vi "String.Validate IP Address String.vi"(11 "IP Address":string) -> (3 "Valid":bool)   [LabVIEW 2019]
panel:
  out "Val 4":i32
  out "Val 3":i32
  out "Val 2":i32
  out "Val 1":i32
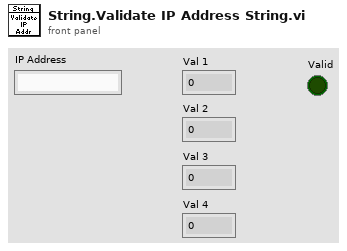
[diagram p1: front panel]
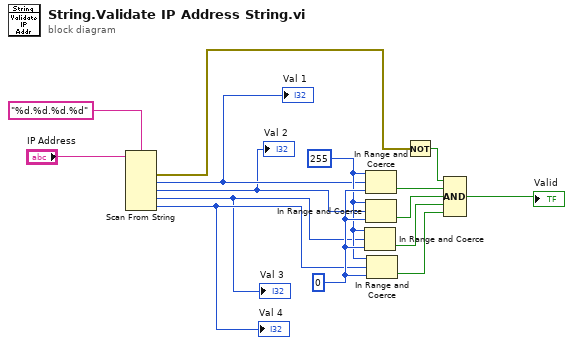
[diagram p0: block diagram]
diagram:
  w13 = 0
  w12 = 255
  n1 = Scan From String(format string="%d.%d.%d.%d", input string="IP Address") -> (error out=w1:errorcluster, output 1=w4:i32, output 2=w3:i32, output 3=w5:i32, output 4=w6:i32)  [unwired: 6 in, 2 out]
  "Val 1" <- w4
  "Val 2" <- w3
  "Val 3" <- w5
  "Val 4" <- w6
  n2 = In Range and Coerce(upper limit=w12, x=w5, lower limit=w13) -> (In Range?=w9:bool)  [unwired: 1 out]
  n3 = In Range and Coerce(upper limit=w12, x=w4, lower limit=w13) -> (In Range?=w11:bool)  [unwired: 1 out]
  n4 = In Range and Coerce(upper limit=w12, x=w3, lower limit=w13) -> (In Range?=w10:bool)  [unwired: 1 out]
  n5 = In Range and Coerce(upper limit=w12, x=w6, lower limit=w13) -> (In Range?=w8:bool)  [unwired: 1 out]
  n6 = Not(x=w1) -> (.not. x?=w2:bool)
  n7 = Compound Arithmetic op=AND(w2, w11, w10, w9, w8) -> (→"Valid":bool)
